vi "DBL To I16.vi"(10 "Audio Data (1D DBL)":dbl[](array[numeric]), 11 "Audio Data (2D DBL)":dbl[][](array[numeric])) -> (2 "Audio Data (1D I16)":i16[](array[numeric]), 3 "Audio Data (2D I16)":i16[][](array[numeric]))   [LabVIEW 2018, in "Audio Processing.lvlib"]
doc: "Converts audio in DBL format (range -1 to 1) to I16 (range -32768 to 32767).\n\nWire 1D array for single channel audio, or 2D array for multi-channel audio."
uses:
  Audio Processing.lvlib
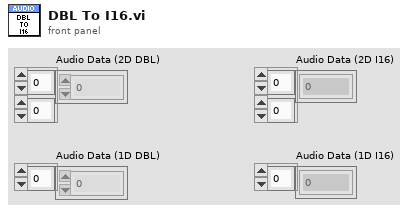
[diagram p1: front panel]
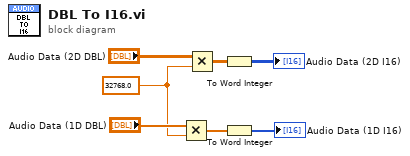
[diagram p0: block diagram]
diagram:
  w3 = 32768.0
  n1 = Multiply(x="Audio Data (1D DBL)", y=w3) -> (x*y=w2:dbl[])
  n2 = Multiply(x="Audio Data (2D DBL)", y=w3) -> (x*y=w6:dbl[][])
  n3 = To Word Integer(number=w6) -> (16bit integer=→"Audio Data (2D I16)":i16[][])
  n4 = To Word Integer(number=w2) -> (16bit integer=→"Audio Data (1D I16)":i16[])
